vi "Set Hardware Configuration File Path.vi"(8 "error in":errorcluster, 9 "Path":path, 11 "Configuration files Ref":T1 format="%.0x") -> (0 "error out":errorcluster, 3 "Configuration files Ref out":T1 format="%.0x")   [LabVIEW 2020, in "Ballard ARINC 429 Scripting.lvlib"]
uses:
  Ballard ARINC 429 Scripting.lvlib
  <vilib>/NI VeriStand/Custom Device API/Custom Device Item Ref.ctl
  Constants.vi
  <vilib>/NI VeriStand/Custom Device API/Set Item Property (Path).vi
  <vilib>/NI VeriStand/Custom Device API/Custom Device API.lvlib
  System Explorer/Implementation/Implementation.lvlib
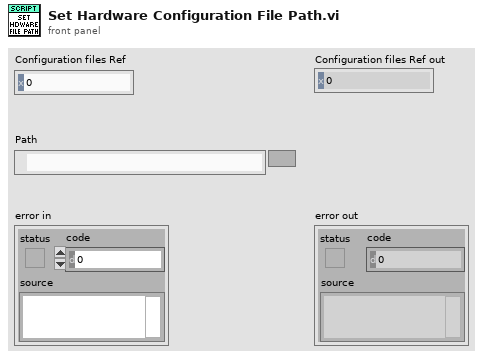
[diagram p1: front panel]
types:
  T1 = typedef "Custom Device API.lvlib/Custom Device Item Ref.ctl" = u64
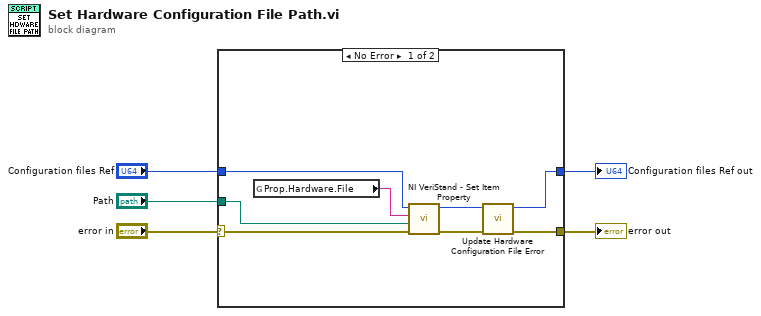
[diagram p0: block diagram]
diagram:
  n1 = case shown="No Error" "error in" {
    selector: "error in" -> [w12 w15]
    tunnel: "Configuration files Ref" -> [w13 w14]
    tunnel: [w6 w15] -> w4
    tunnel: [w8 w14] -> w2
    tunnel: "Path" -> [w10 _]
    frame No Error {
      n2 = global read "Constants.vi" "Prop.Hardware.File"() -> (w11:string)
      n3 = call-poly <vilib>:"NI VeriStand - Set Item Property.vi"("error in (no error)"=w12, "Value"=w10, "Property Name"=w11, "Item Ref in"=w13) -> ("error out"=w7:errorcluster, "Item Ref out"=w9:T1)  [unwired: 5 in, 1 out]
      n4 = call "Update Hardware Configuration File Error.vi"("error in"=w7, "Configuration files Ref"=w9) -> ("error out"=w6:errorcluster, "Configuration files Ref out"=w8:T1)  [unwired: 8 in]
    }
    frame Error {
    }
  }
  "error out" <- w4
  "Configuration files Ref out" <- w2
